vi "trash_Read Benchmarks.vi"(11 "CIF_NIChn_Fifo_DAQ in":refnum<class "CIF_NIChn_Fifo_DAQ.lvclass">) -> (0 "Channel Avg":dbl, 1 "Channel Max":i64, 2 "Flatten Avg":dbl, 3 "Flatten Max":i64)   [LabVIEW 2021]
uses:
  <vilib>/CIF Foundation/CIF Utilities/Statistics/I64/Stats_I64_CIF_U.lvclass
  CIF_NIChn_Fifo_DAQ.lvclass
  D:/dev/Packages/Channel_Manager/src/CIF_NIChn/NIChn/CIF_NIChn.lvclass
  D:/dev/Packages/Channel_Manager/src/CIFChannels/CIFChannels.lvclass
  D:/dev/Packages/Channel_Manager/src/CIF_NIChn/FIFO_DAQ/CIF_NIChn_Fifo_DAQ.lvclass
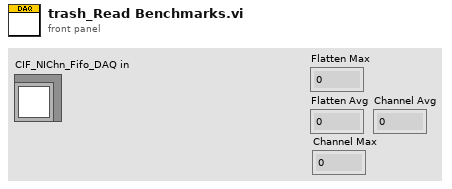
[diagram p1: front panel]
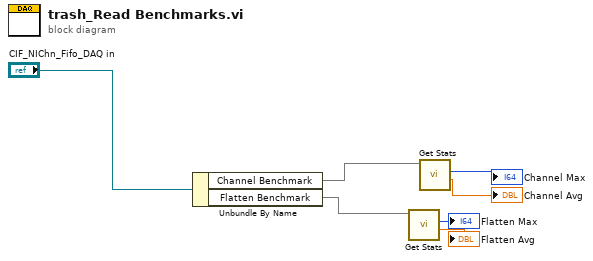
[diagram p0: block diagram]
diagram:
  n1 = Unbundle By Name("CIF_NIChn_Fifo_DAQ in") -> ("Channel Benchmark"=w5, "Flatten Benchmark"=w6)
  n2 = call <vilib>:"Get Stats.vi"("Stats_I64_CIF_U in"=w6) -> ("Average"=→"Flatten Avg":dbl, "Max"=→"Flatten Max":i64)  [unwired: 6 in, 3 out]
  n3 = call <vilib>:"Get Stats.vi"("Stats_I64_CIF_U in"=w5) -> ("Average"=→"Channel Avg":dbl, "Max"=→"Channel Max":i64)  [unwired: 6 in, 3 out]
